vi "Begin Communicate Stream.vi"(6 "contextId":T1, 8 "error in":errorcluster, 9 "timeout (ms)":i32=-1, 10 "Request Data":T2, 11 "gRPC ID":T1) -> (0 "error out":errorcluster, 2 "Call Id Out":T1, 3 "gRPC ID out":T1)   [LabVIEW 2021, in "Demo_client.lvlib"]
uses:
  Demo_client.lvlib
  <vilib>/gRPC/LabVIEW gRPC Library/Shared/grpcId.ctl
  RPC Messages/Communication_ControlStream.ctl
  59bd46bd-855a-43b3-a0b3-6a244c6a481b.vi
  <vilib>/gRPC/LabVIEW gRPC Library/Shared/TranslateGrpcError.vi
  <vilib>/gRPC/LabVIEW gRPC Library/Server API/Server/Get Server DLL Path.vi
  <vilib>/Utility/error.llb/Error Cluster From Error Code.vi
  <vilib>/Utility/error.llb/Simple Error Handler.vi
  <vilib>/gRPC/LabVIEW gRPC Library/grpc-lvsupport-release.lvlib
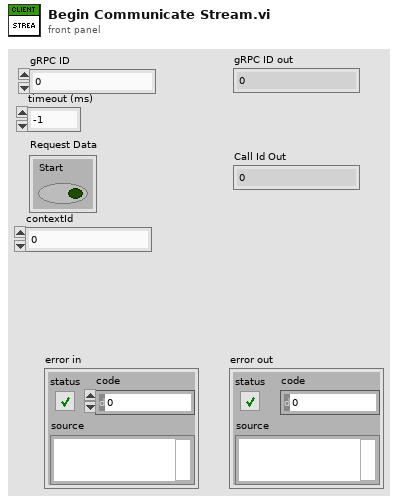
[diagram p1: front panel]
types:
  T1 = typedef "grpc-lvsupport-release.lvlib/grpcId.ctl" = u64
  T2 = typedef "Demo_client.lvlib/Communication_ControlStream.ctl" = cluster{"Start":bool}
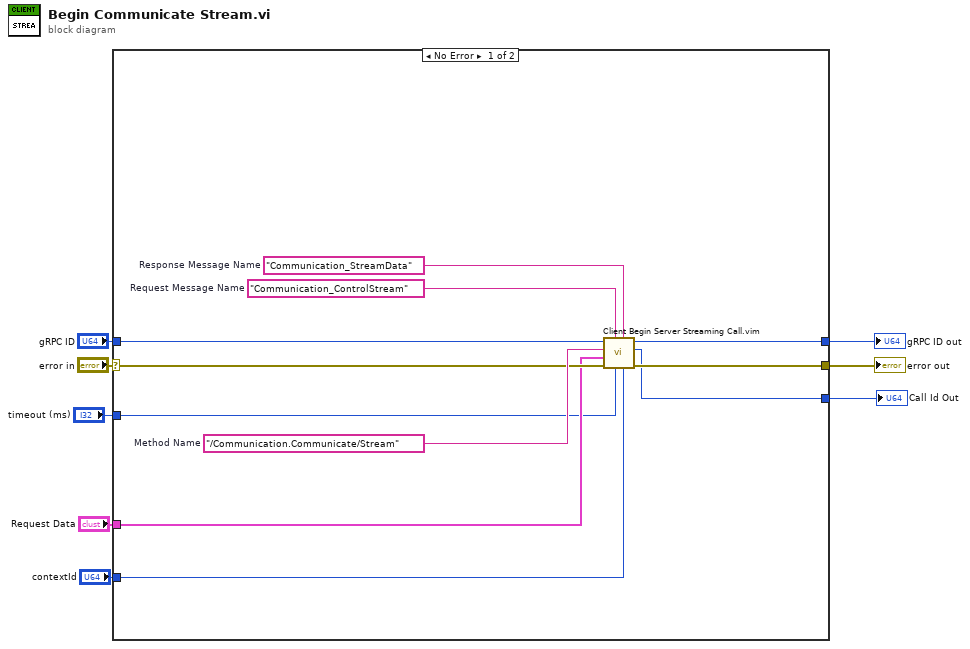
[diagram p0: block diagram]
diagram:
  n1 = case shown="No Error" "error in" {
    selector: "error in" -> [w16 w20]
    tunnel: [w15 w20] -> w7
    tunnel: "gRPC ID" -> [w14 w21]
    tunnel: [w13 w21] -> w5
    tunnel: [w12 _] -> w4
    tunnel: "Request Data" -> [w11 _]
    tunnel: "timeout (ms)" -> [w10 _]
    tunnel: "contextId" -> [w9 _]
    frame No Error {
      w17 = "Communication_StreamData"  # Response Message Name
      w18 = "Communication_ControlStream"  # Request Message Name
      w19 = "/Communication.Communicate/Stream"  # Method Name
      n2 = call "Client Begin Server Streaming Call.vim"("contextId"=w9, "Response Message Name"=w17, "timeout (ms)"=w10, "Request Message Name"=w18, "error in"=w16, "Request Data"=w11, "Method Name"=w19, "ClientID in"=w14) -> ("error out"=w15:errorcluster, "Call ID out"=w12:u64, "ClientID out"=w13:u64)  [unwired: 1 in]
    }
    frame Error {
    }
  }
  "error out" <- w7
  "gRPC ID out" <- w5
  "Call Id Out" <- w4
